vi "LFU Retrieve File Handle__ogtk.vi"(4 "error in (no error)":errorcluster, 7 "file refnum":refnum<file>) -> (0 "error out":errorcluster, 3 "handle out":u32)   [LabVIEW 2012]
doc: "Low level utility function to retrieve the platform API specific file handle from a LabVIEW file handle."
panel:
  # "LFU Retrieve File Handle.vi\n\nPlease visit http://www.OpenG.org to learn about the\nOpen Source LabVIEW software movement.\n\nNOTICE -- YOU MUST LEAVE THIS NOTICE IN PLACE.  PER THE TERMS OF THE LICENSE BELOW, YOU MAY SUBLICENSE THIS SOFTWARE \nIN ANY WAY THAT DOES NOT CONFLICT WITH THIS LICENSE.\n\n### BSD License (http://www.opensource.org/licenses/bsd-license.php) Begin ###\n\nCopyright (c) 2003, Rolf Kalbermatter <rolf.kalbermatter@citeng.com>\n\nAll rights reserved.\n\nRedistribution and use in source and binary forms, with or without modification, are permitted provided that the following conditions are met:\n\n    * Redistributions of source code must retain the above copyright notice, this list of conditions and the following disclaimer.\n    * Redistributions in binary form must reproduce the above copyright notice, this list of conditions and the following disclaimer in the \n       documentation and/or other materials provided with the distribution.\n    * Neither the name of SciWare, James Kring, Inc., nor the names of its contributors may be used to endorse or promote products derived \n       from this software without specific prior written permission.\n\nTHIS SOFTWARE IS PROVIDED BY THE COPYRIGHT HOLDERS AND CONTRIBUTORS \"AS IS\" AND ANY EXPRESS OR IMPLIED WARRANTIES, \nINCLUDING, BUT NOT LIMITED TO, THE IMPLIED WARRANTIES OF MERCHANTABILITY AND FITNESS FOR A PARTICULAR PURPOSE ARE \nDISCLAIMED. IN NO EVENT SHALL THE COPYRIGHT OWNER OR CONTRIBUTORS BE LIABLE FOR ANY DIRECT, INDIRECT, INCIDENTAL,\n SPECIAL, EXEMPLARY, OR CONSEQUENTIAL DAMAGES (INCLUDING, BUT NOT LIMITED TO, PROCUREMENT OF SUBSTITUTE GOODS OR \nSERVICES; LOSS OF USE, DATA, OR PROFITS; OR BUSINESS INTERRUPTION) HOWEVER CAUSED AND ON ANY THEORY OF LIABILITY, \nWHETHER IN CONTRACT, STRICT LIABILITY, OR TORT (INCLUDING NEGLIGENCE OR OTHERWISE) ARISING IN ANY WAY OUT OF THE USE \nOF THIS SOFTWARE, EVEN IF ADVISED OF THE POSSIBILITY OF SUCH DAMAGE.\n\n### BSD License End ###"
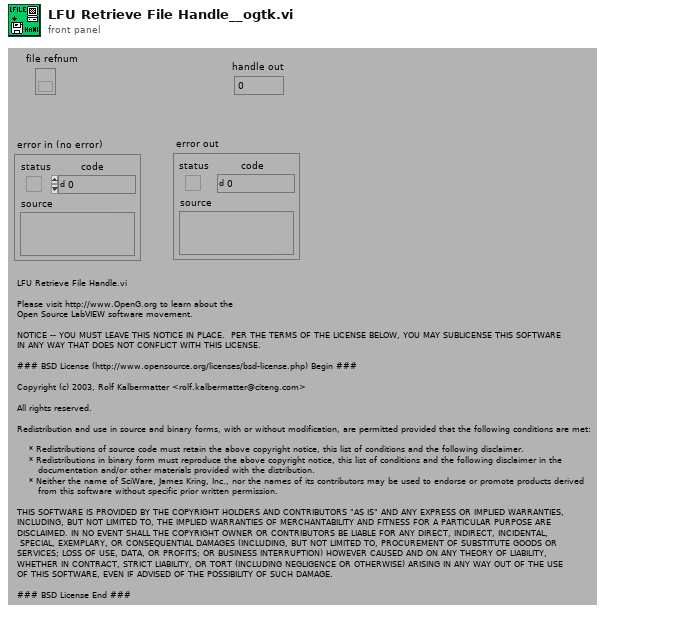
[diagram p1: front panel]
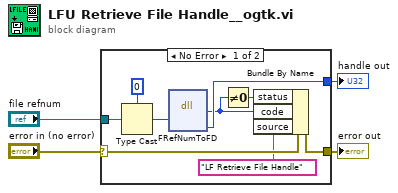
[diagram p0: block diagram]
diagram:
  n1 = case shown="No Error" "error in (no error)" {
    selector: "error in (no error)" -> [w13 w15]
    tunnel: [w9 u32 0 ("fd")] -> w4
    tunnel: "file refnum" -> [w6 _]
    tunnel: [w12 w15] -> w1
    frame No Error {
      n2 = Type Cast(type=u32 0 ("refNum"), x=w6) -> (*(type *) &x=w5:u32)
      n3 = dll-call lib="LabVIEW" fn="FRefNumToFD"("refNum"=w5) -> (w7:i32, "fd"=w9:u32)  [unwired: 5 in, 2 out]
      n4 = Not Equal To 0?(x=w7) -> (x != 0?=w8:bool)
      n5 = Bundle By Name(cluster=w13, "status"=w8, "code"=w7, "source"="LF Retrieve File Handle") -> (w12:errorcluster)
    }
    frame Error {
    }
  }
  "handle out" <- w4
  "error out" <- w1
